vi "Interpolate_Align_Corners=False.vi"(10 "target Dims":i32[](array[numeric]), 11 "Array":sgl[][][](array[numeric])) -> (3 "Out":sgl[][][](array[numeric]), 5 "time elapsed":dbl)   [LabVIEW 2020]
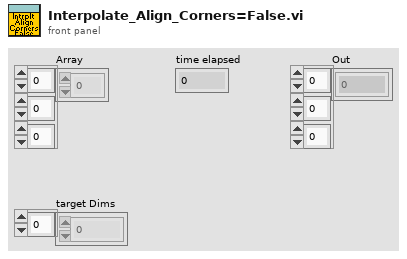
[diagram p1: front panel]
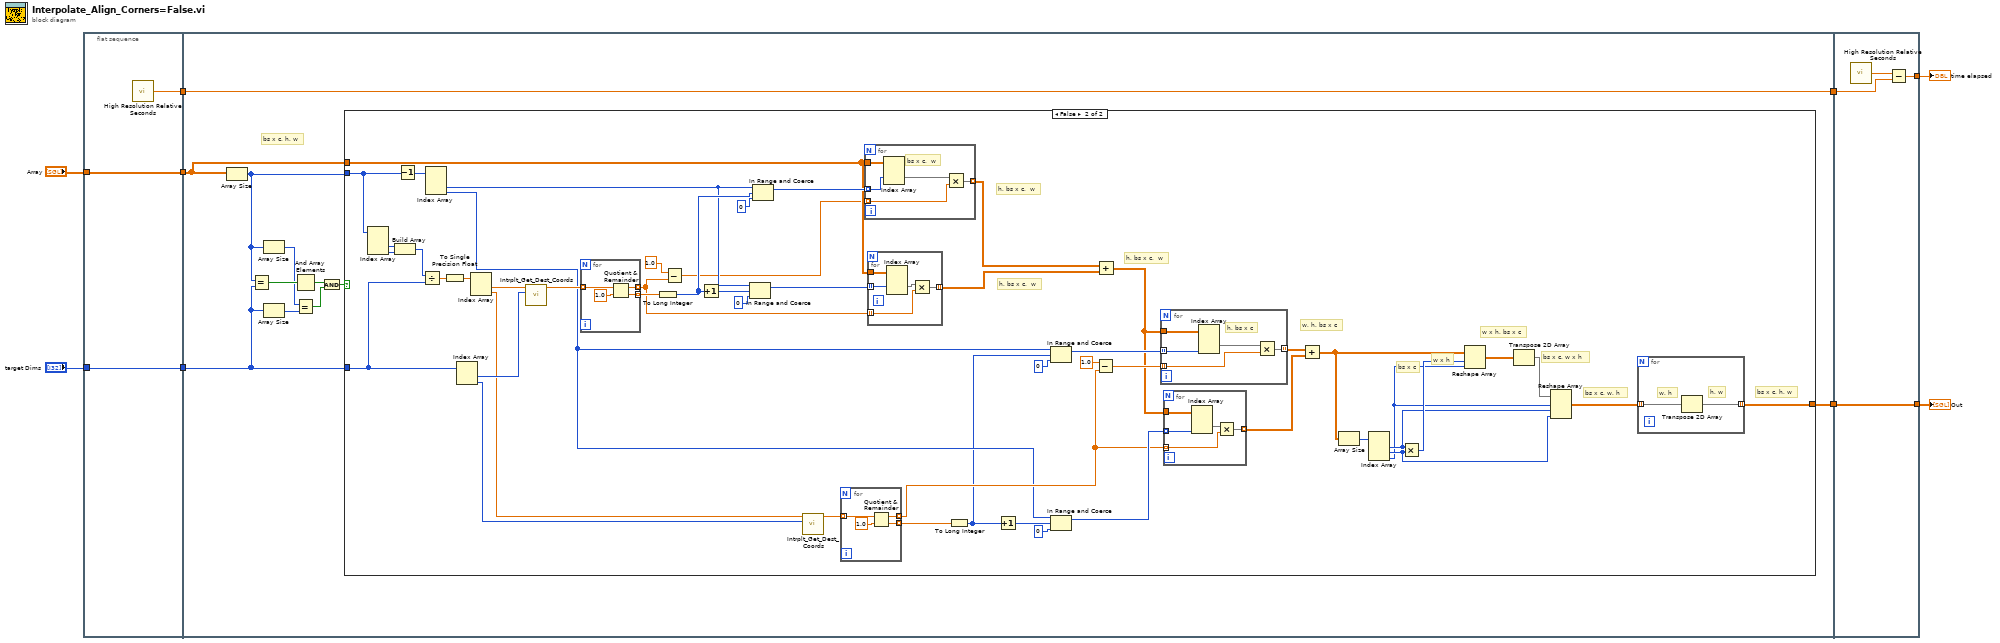
[diagram p0: block diagram]
diagram:
  n1 = flat-sequence {
    tunnel: "target Dims" -> [w11]
    tunnel: "Array" -> [w12]
    tunnel: [w12] -> w6
    tunnel: [w11] -> w5
    tunnel: [w10] -> w2
    tunnel: w6 -> [w22]
    tunnel: w5 -> [w18]
    tunnel: [w23] -> w4
    tunnel: [w13] -> w3
    tunnel: w2 -> [w13]
    tunnel: [w110] -> w9
    tunnel: w4 -> [w110]
    tunnel: w3 -> [w108]
    tunnel: [w107] -> w1
    frame #0 {
      n2 = call <vilib>:"High Resolution Relative Seconds.vi"() -> ("relative seconds"=w10:dbl)
    }
    frame #1 {
      # "bs x c, h, w"
      n3 = Array Size(array=w22) -> (size(s)=w19:i32[])
      n4 = Equal?(x=w19, y=w18) -> (x = y?=w21:bool[])
      n5 = Array Size(array=w19) -> (size(s)=w16:i32)
      n6 = Array Size(array=w18) -> (size(s)=w17:i32)
      n7 = And Array Elements(Boolean array=w21) -> (logical AND=w20:bool)
      n8 = Equal?(x=w16, y=w17) -> (x = y?=w14:bool)
      n9 = And(x=w20, y=w14) -> (x .and. y?=w15:bool)
      n10 = case shown="False" w15 {
        tunnel: w18 -> [_ w75]
        tunnel: [w24 w44] -> w23
        tunnel: w19 -> [_ w43]
        tunnel: w22 -> [w24 w37]
        frame True {
        }
        frame False {
          # "bs x c, h, w"
          # "bs x c, w, h"
          # "bs x c, w x h"
          # "w x h, bs x c"
          # "bs x c"
          # "w x h"
          # "w, h, bs x c"
          # "h, bs x c,  w"
          # "h, bs x c,  w"
          # "h, bs x c,  w"
          n11 = Index Array(array=w43) -> (element #2=w42:i32, element #3=w41:i32)  [unwired: 3 in, 1 out]
          n12 = Build Array(w42, w41) -> (w40:i32[])
          n13 = Decrement(x=w43) -> (x-1=w68:i32[])
          n14 = Divide(x=w40, y=w75) -> (x/y=w74:dbl[])
          n15 = Index Array(array=w68) -> (element #2=w64:i32, element #3=w45:i32)  [unwired: 3 in, 1 out]
          n16 = To Single Precision Float(number=w74) -> (single precision float=w26:sgl[])
          n17 = Index Array(array=w75) -> (element #1=w76:i32, element #2=w57:i32)  [unwired: 2 in]
          n18 = Index Array(array=w26) -> (element #1=w73:sgl, element #2=w58:sgl)  [unwired: 2 in]
          n19 = call "Intrplt_Get_Dest_Coords.vi"("Dim"=w76, "Step"=w73) -> ("Coords"=w72:sgl[])  [unwired: 9 in]
          n20 = for {
            tunnel: w72 -> [w101] mode=indexing
            tunnel: [w98] -> w61 mode=indexing
            tunnel: [w99] -> w71 mode=indexing
            n21 = Quotient & Remainder(x=w101, y=sgl 1.0) -> (x-y*floor(x/y)=w98:sgl, floor(x/y)=w99:sgl)
          }
          n22 = To Long Integer(number=w71) -> (32bit integer=w67:i32[])
          n23 = Subtract(x=sgl 1.0, y=w61) -> (x-y=w28:sgl[])
          n24 = Increment(x=w67) -> (x+1=w65:i32[])
          n25 = In Range and Coerce(upper limit=w64, x=w65, lower limit=0) -> (coerced(x)=w60:i32[])  [unwired: 1 out]
          n26 = In Range and Coerce(upper limit=w64, x=w67, lower limit=0) -> (coerced(x)=w70:i32[])  [unwired: 1 out]
          n27 = call "Intrplt_Get_Dest_Coords.vi"("Dim"=w57, "Step"=w58) -> ("Coords"=w46:sgl[])  [unwired: 9 in]
          n28 = for {
            tunnel: w46 -> [w97] mode=indexing
            tunnel: [w94] -> w54 mode=indexing
            tunnel: [w95] -> w47 mode=indexing
            n29 = Quotient & Remainder(x=w97, y=sgl 1.0) -> (x-y*floor(x/y)=w94:sgl, floor(x/y)=w95:sgl)
          }
          n30 = for {
            tunnel: w37 -> [w105]
            tunnel: w70 -> [w102] mode=indexing
            tunnel: [w104] -> w63 mode=indexing
            tunnel: w28 -> [w103] mode=indexing
            # "bs x c,  w"
            n31 = Index Array(array=w105, index (dim 1)=w102) -> (element=w106:sgl[][])  [unwired: 2 in]
            n32 = Multiply(x=w106, y=w103) -> (x*y=w104:sgl[][])
          }
          n33 = for {
            tunnel: w37 -> [w82]
            tunnel: w60 -> [w79] mode=indexing
            tunnel: [w81] -> w59 mode=indexing
            tunnel: w61 -> [w80] mode=indexing
            n34 = Index Array(array=w82, index (dim 1)=w79) -> (element=w83:sgl[][])  [unwired: 2 in]
            n35 = Multiply(x=w83, y=w80) -> (x*y=w81:sgl[][])
          }
          n36 = To Long Integer(number=w47) -> (32bit integer=w27:i32[])
          n37 = Increment(x=w27) -> (x+1=w51:i32[])
          n38 = In Range and Coerce(upper limit=w45, x=w27, lower limit=0) -> (coerced(x)=w48:i32[])  [unwired: 1 out]
          n39 = In Range and Coerce(upper limit=w45, x=w51, lower limit=0) -> (coerced(x)=w55:i32[])  [unwired: 1 out]
          n40 = Subtract(x=sgl 1.0, y=w54) -> (x-y=w53:sgl[])
          n41 = Add(x=w63, y=w59) -> (x+y=w39:sgl[][][])
          n42 = for {
            tunnel: w39 -> [w87]
            tunnel: w48 -> [w84] mode=indexing
            tunnel: [w86] -> w38 mode=indexing
            tunnel: w53 -> [w85] mode=indexing
            # "h, bs x c"
            n43 = Index Array(array=w87, index (dim 2)=w84) -> (element=w88:sgl[][])  [unwired: 2 in]
            n44 = Multiply(x=w88, y=w85) -> (x*y=w86:sgl[][])
          }
          n45 = for {
            tunnel: w39 -> [w92]
            tunnel: w55 -> [w89] mode=indexing
            tunnel: [w91] -> w56 mode=indexing
            tunnel: w54 -> [w90] mode=indexing
            n46 = Index Array(array=w92, index (dim 2)=w89) -> (element=w93:sgl[][])  [unwired: 2 in]
            n47 = Multiply(x=w93, y=w90) -> (x*y=w91:sgl[][])
          }
          n48 = Add(x=w38, y=w56) -> (x+y=w36:sgl[][][])
          n49 = Array Size(array=w36) -> (size(s)=w35:i32[])
          n50 = Index Array(array=w35) -> (element #1=w31:i32, element #2=w30:i32, element #3=w25:i32)  [unwired: 3 in]
          n51 = Multiply(x=w31, y=w30) -> (x*y=w34:i32)
          n52 = Reshape Array(w36, w34, w25) -> (w33:sgl[][])
          n53 = Transpose 2D Array(2D array=w33) -> (transposed array=w32:sgl[][])
          n54 = Reshape Array(w32, w25, w31, w30) -> (w29:sgl[][][])
          n55 = for {
            tunnel: w29 -> [w78] mode=indexing
            tunnel: [w77] -> w44 mode=indexing
            # "h, w"
            # "w, h"
            n56 = Transpose 2D Array(2D array=w78) -> (transposed array=w77:sgl[][])
          }
        }
      }
    }
    frame #2 {
      n57 = call <vilib>:"High Resolution Relative Seconds.vi"() -> ("relative seconds"=w109:dbl)
      n58 = Subtract(x=w109, y=w108) -> (x-y=w107:dbl)
    }
  }
  "Out" <- w9
  "time elapsed" <- w1
